vi "OCT with Classes.vi"() -> ()   [LabVIEW 2014]
doc: "I. Description:\nThis example demonstrates how to acquire a continuous amount of data (Waveform) using the DAQ device's internal clock.\n\nII. Instructions for Running:\n1. Create an analog input voltage channel.\n2. Set the rate for the sample clock. Additionally, define the sample mode to be continuous.\n3. Call the Start VI to start the acquisition.\n4. Read the waveform data in a loop until the user hits the stop button or an error occurs.\nNote: This example reads data from one or more channels and returns an array of data. Use the Index Array function to access an individual channel of data.\n5. Call the Clear Task VI to clear the Task.\n6. Use the popup dialog box to display an error if any.\n\nIV. I/O Connections Overview:\nMake sure your signal input terminal matches the Physical Channel I/O Control. For further connection information, refer to your hardware reference manual."
uses:
  Type Defs/OCT DAQ Channel Data Type.ctl
  Type Defs/OCT Hardware States.ctl
  Classes/Galvo/Scanning Cluster.ctl
  Classes/UT OCT Classes.ctl
  Classes/DAQ/ATS660/ATS660 Class.lvclass
  Classes/Galvo/NI Galvo/NI Galvo.lvclass
  Processing Class/Intensity/Intensity Processing.lvclass
  Classes/Laser/Santec/Santec.lvclass
  Classes/DAQ Control Functional Global States.ctl
  Signal Processing/Display Raw Data states.ctl
  DAQ Status States.ctl
  Signal Processing/processing_states.ctl
  Classes/Galvo/Galvo.lvclass
panel:
  out "Single A-Scan":u16[](graph)
  in  "Scanning Parameters":T1={"Fast Axis Offset"=0.0, "Slow Axis Offset"=0.0, "Slow Axis Amp"=2.0, "Fast Axis Amp"=2.0, "Scan Pattern"=enum."Raster"} {"Fast Axis Amp" max=20 format="%#.2f"; "Slow Axis Amp" max=20 format="%#.2f"; "Slow Axis Offset" max=10 format="%#.2f"; "Fast Axis Offset" max=10 format="%#.2f"}
  out "Log10?":bool
  in  "OCT Hardware States":T2
  out "Background Array":u16[](array[numeric])
  in  "Calibrate":bool
  in  "Save Sweep Button":bool
  in  "Data Format":T3
  in  "Save Sweep":bool
  in  "Stop Button":bool
  out "B-Scans Per Buffer":i32=1
  out "Clock Length":u32=9184
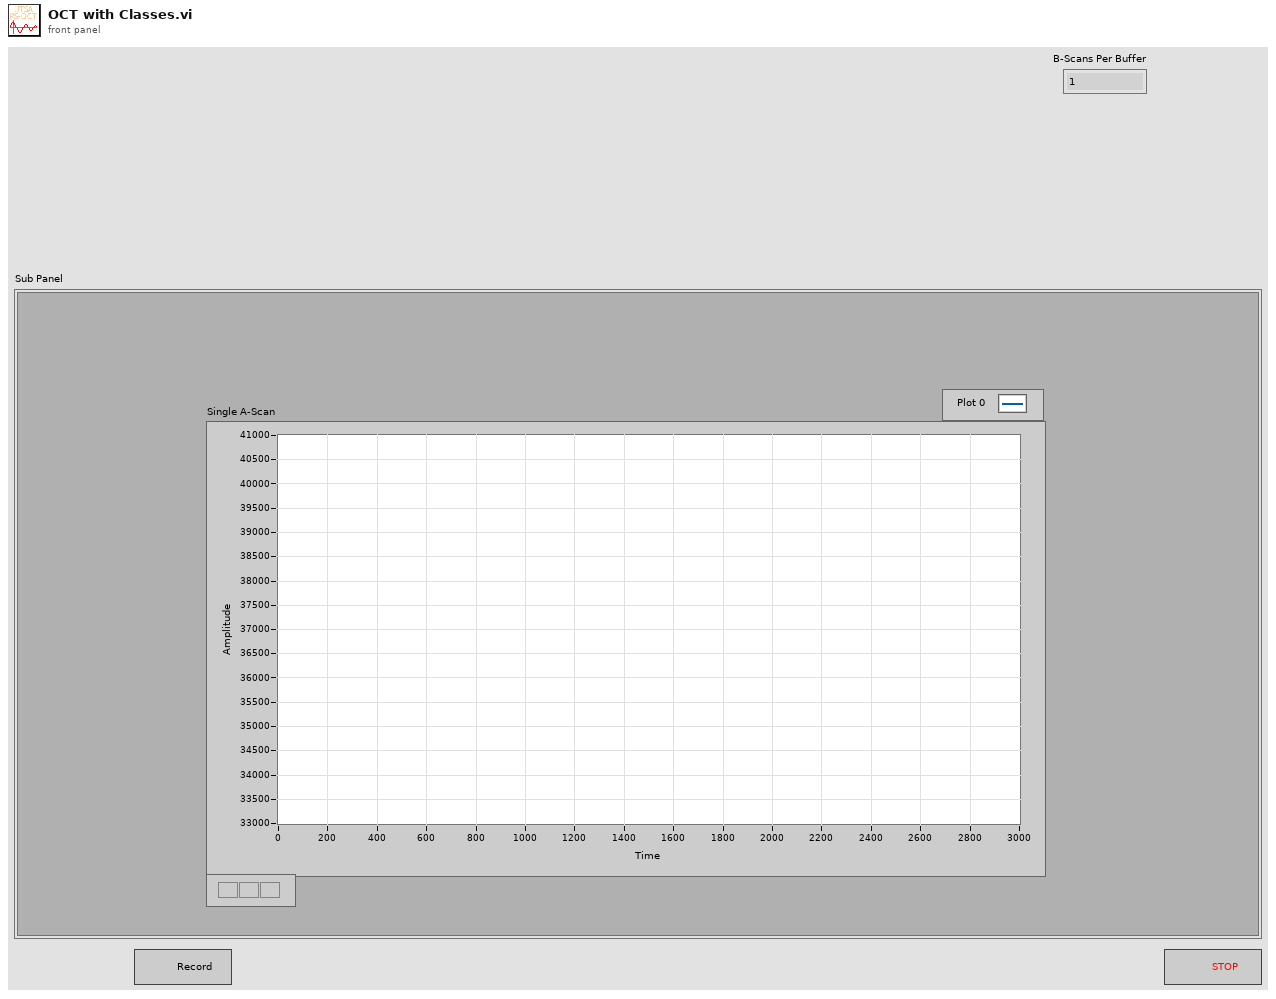
[diagram p1: front panel]
types:
  T1 = typedef "Galvo.lvclass/Scanning Cluster.ctl" = cluster{"Fast Axis Offset":sgl, "Slow Axis Offset":sgl, "Slow Axis Amp":sgl, "Fast Axis Amp":sgl, "Scan Pattern":enum16{"Raster"}}
  T2 = typedef "OCT Hardware States.ctl" = enum16{"Acquire Data", "Initialize Galvos", "Startup", "Reset DAQ", "Background Subtraction", "Acquire Background", "Update DAQ Parameters", "Stop", "Set Clock", "Initialize DAQ", "Set Resampling Array", "Save Sweep", "Configure Laser"}
  T3 = typedef "OCT DAQ Channel Data Type.ctl" = enum16{"Channel 1", "Channel 2", "Channel 1 and 2"}
  T4 = typedef "UT OCT Classes.ctl" = refnum<class "ATS660 Class.lvclass">
  T5 = typedef "DAQ Control Functional Global States.ctl" = enum16{"Status", "Set Processing Finished", "Reset", "Clear", "Set DAQ Finished"}
  T6 = typedef "DAQ Class.lvclass/DAQ Parameters.ctl" = cluster{"Points Per Trigger":u32, "Triggers per Buffer":u32, "Number of Buffers":u32, "Buffers per Transfer":u32, "Trigger Voltage":sgl, "Trigger Source":T7, "Trigger Slope":T8, "Channel":T3, "Clock":T9, "Bits per Sample":dbl, "Range":dbl}
  T7 = typedef "DAQ Class.lvclass/Trigger Source.ctl" = enum16{"External", "Channel A", "Channel B"}
  T8 = typedef "DAQ Class.lvclass/Trigger Slope.ctl" = enum16{"Rising", "Falling"}
  T9 = typedef "DAQ Class.lvclass/Clock Control.ctl" = enum16{"Internal Clock", "External Clock"}
  T10 = typedef "Display Raw Data states.ctl" = enum16{"Add Raw", "Add Processed", "Show"}
  T11 = typedef "DAQ Status States.ctl" = enum16{"Get", "Show"}
  T12 = enum32{"Invalid", "Standard", "Closed", "Hidden", "Minimized", "Maximized"}
  T13 = typedef "processing_states.ctl" = enum16{"Initialize", "Set Background", "Update Imaging Parameters", "Get Queue", "Process Data", "Get Size", "Flush Data", "Set Reample Array", "Get Last Processed BScan", "Shutdown"}
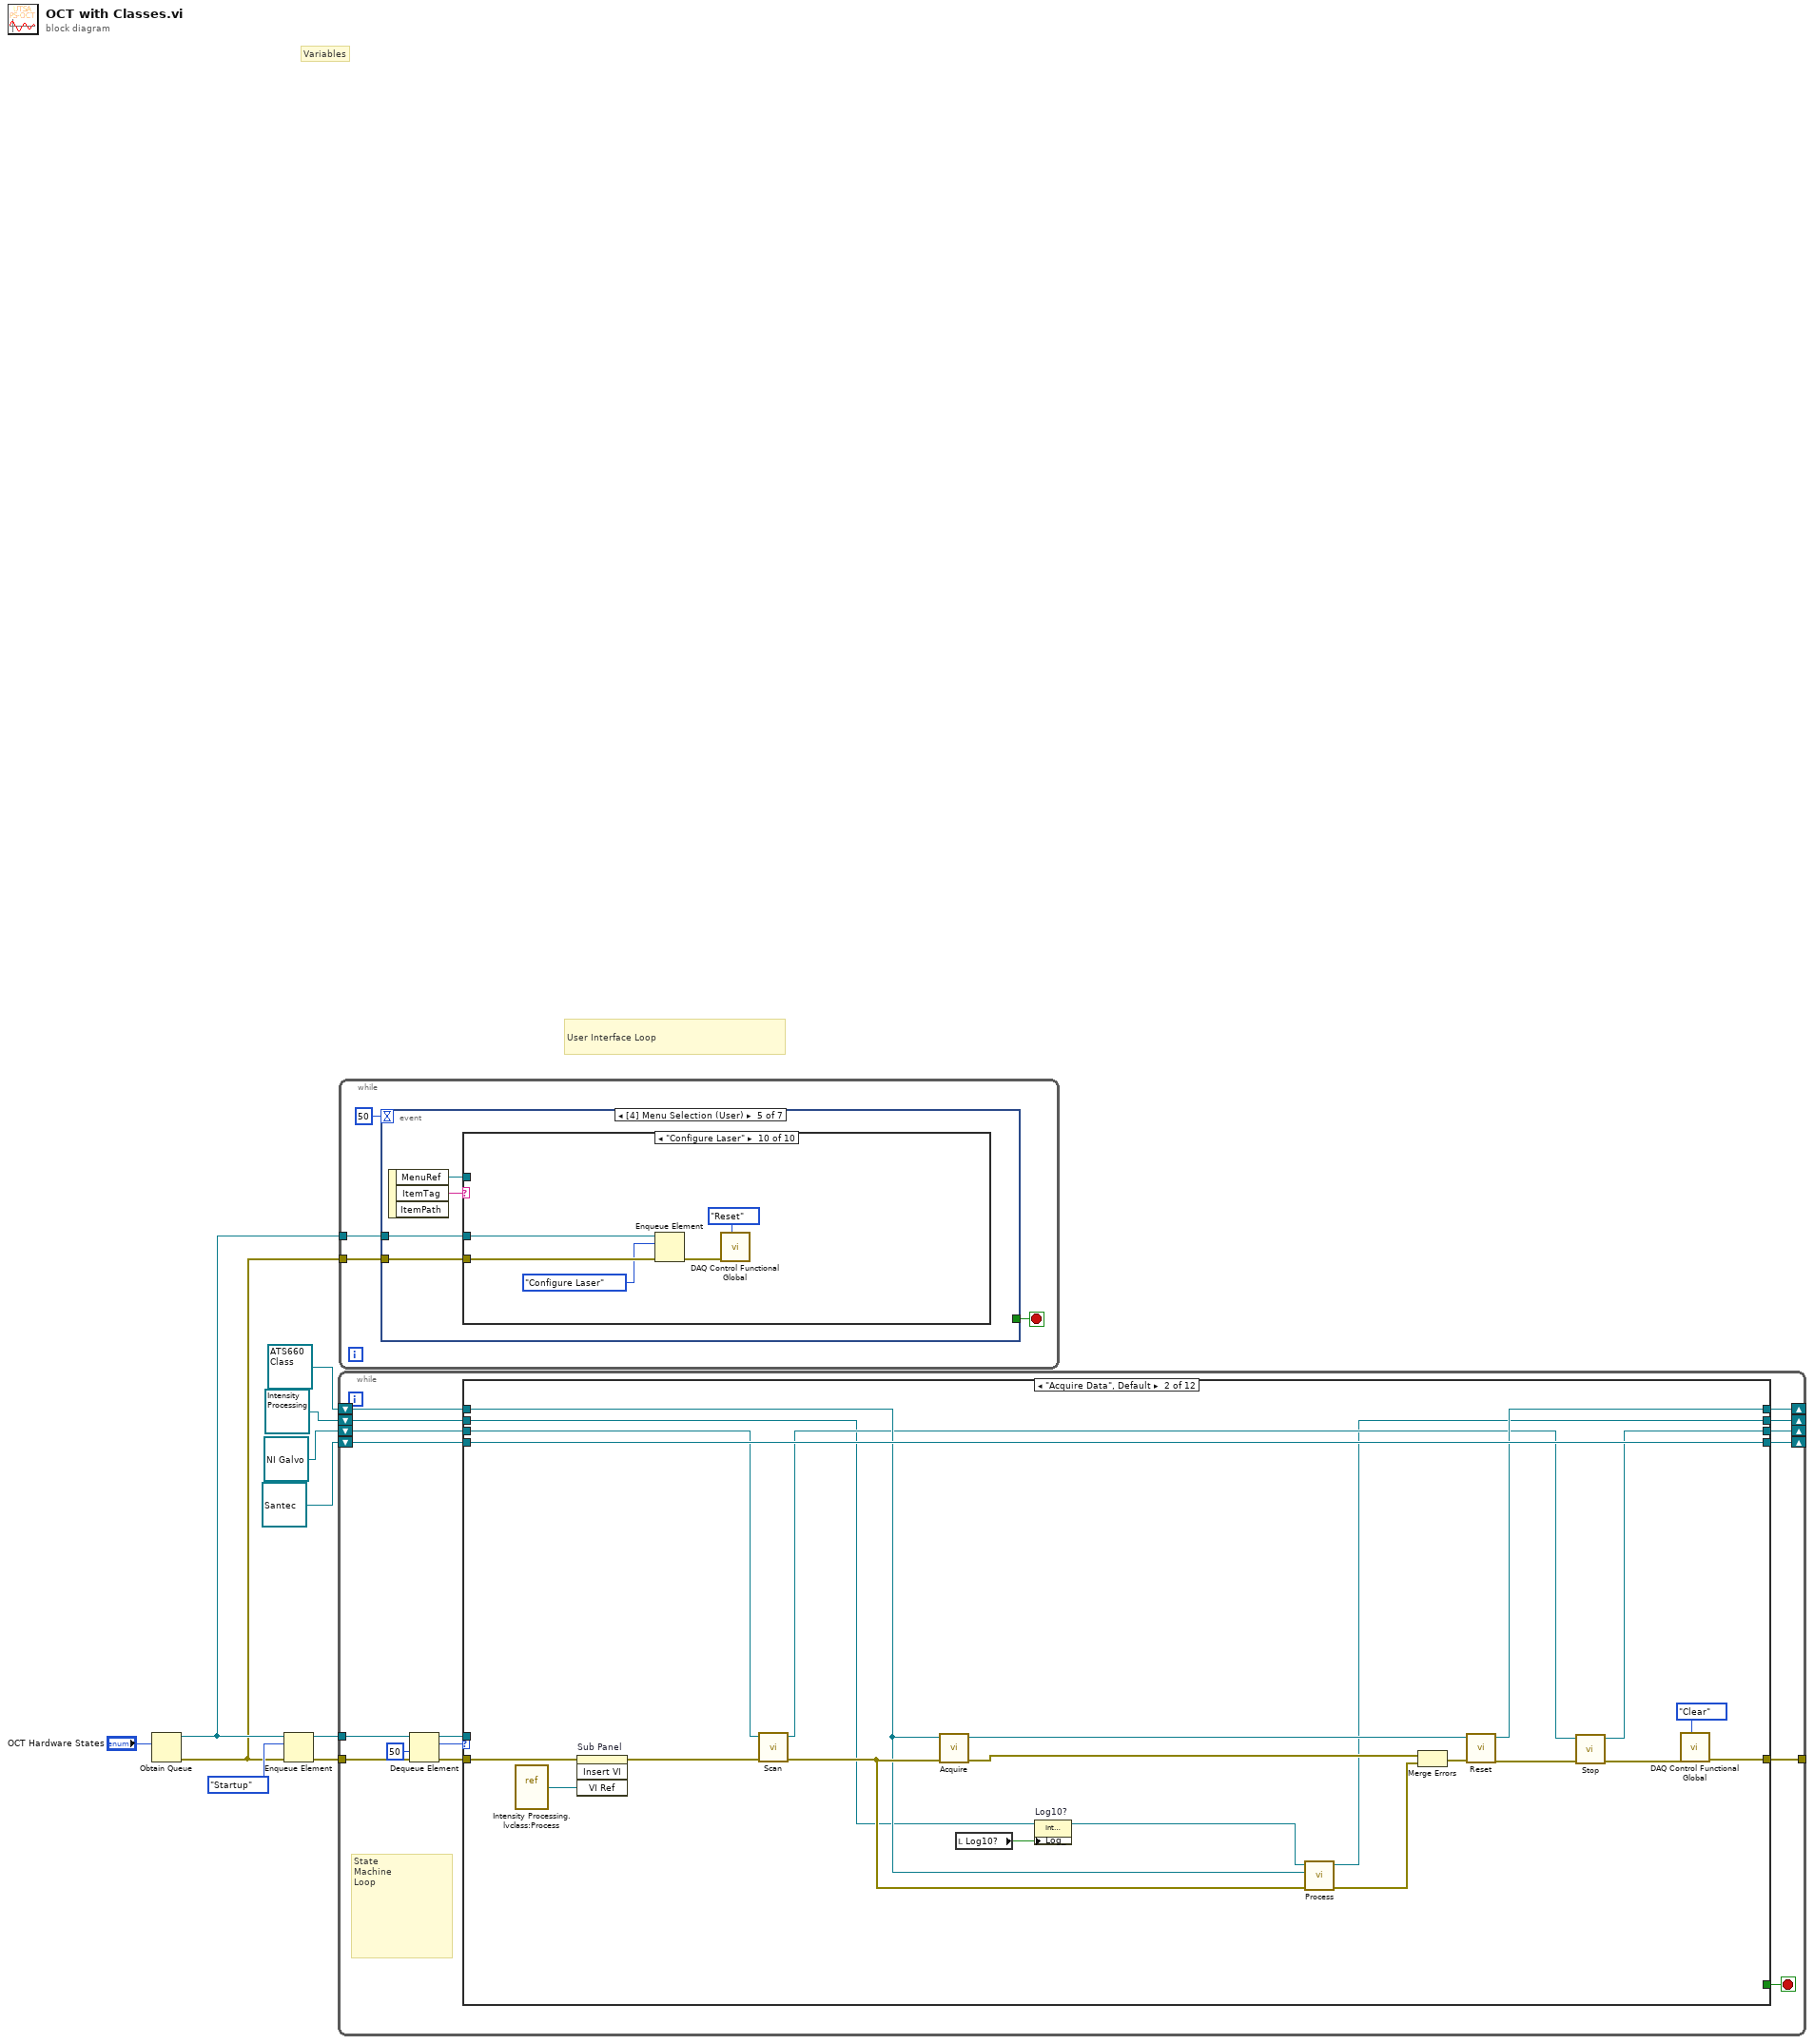
[diagram p0: block diagram]
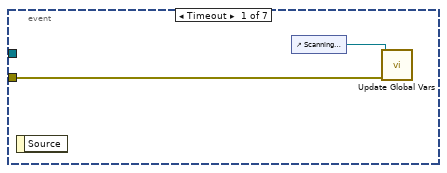
[diagram p2: hidden frame]
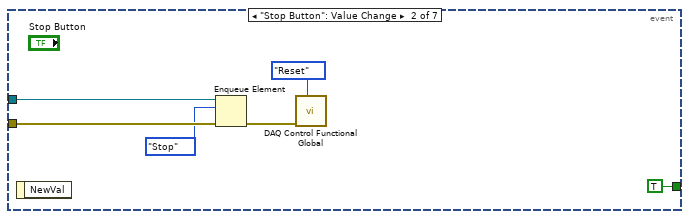
[diagram p3: hidden frame]
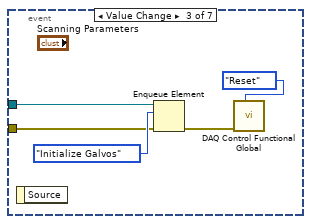
[diagram p4: hidden frame]
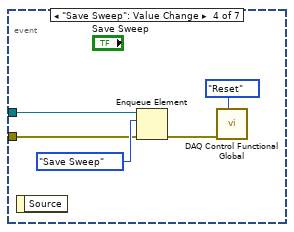
[diagram p5: hidden frame]
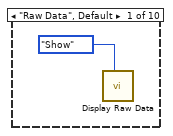
[diagram p6: hidden frame]
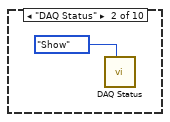
[diagram p7: hidden frame]
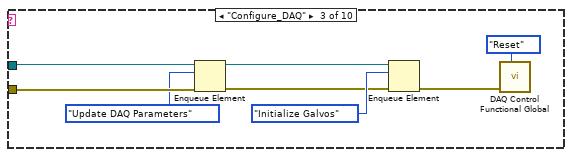
[diagram p8: hidden frame]
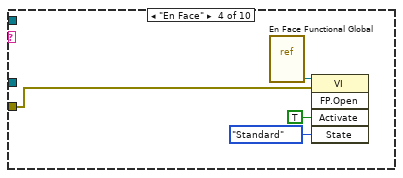
[diagram p9: hidden frame]
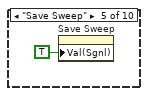
[diagram p10: hidden frame]
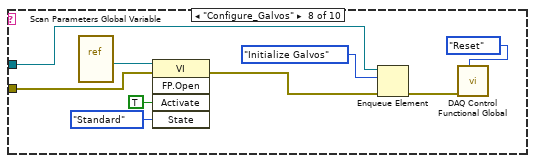
[diagram p13: hidden frame]
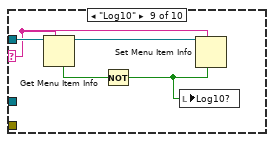
[diagram p14: hidden frame]
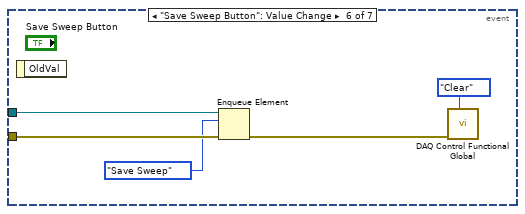
[diagram p15: hidden frame]
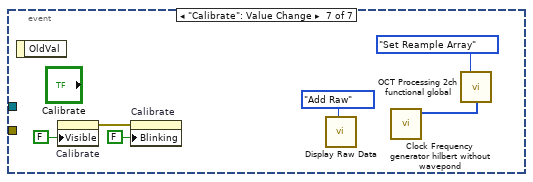
[diagram p16: hidden frame]
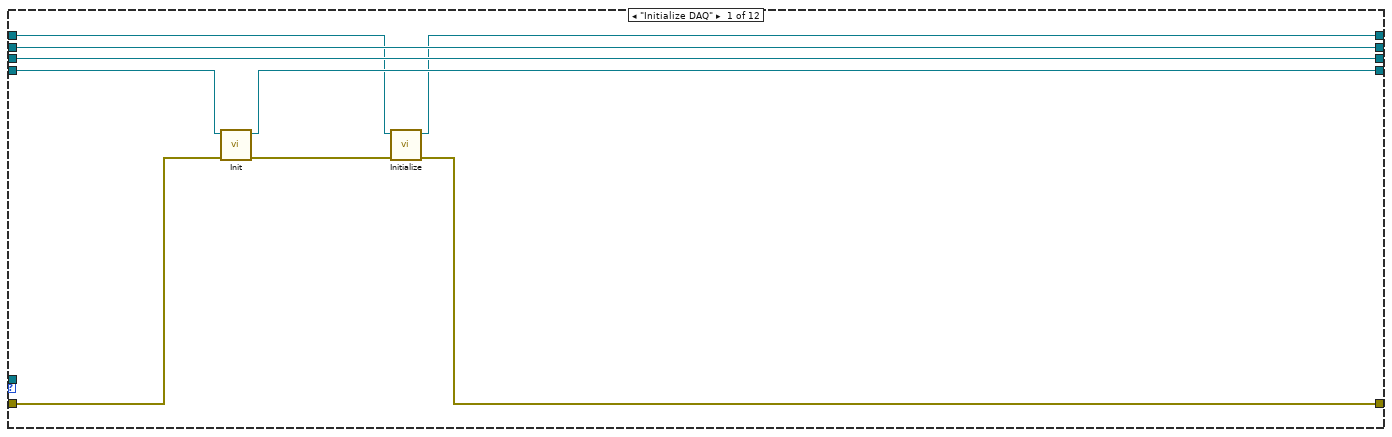
[diagram p17: hidden frame]
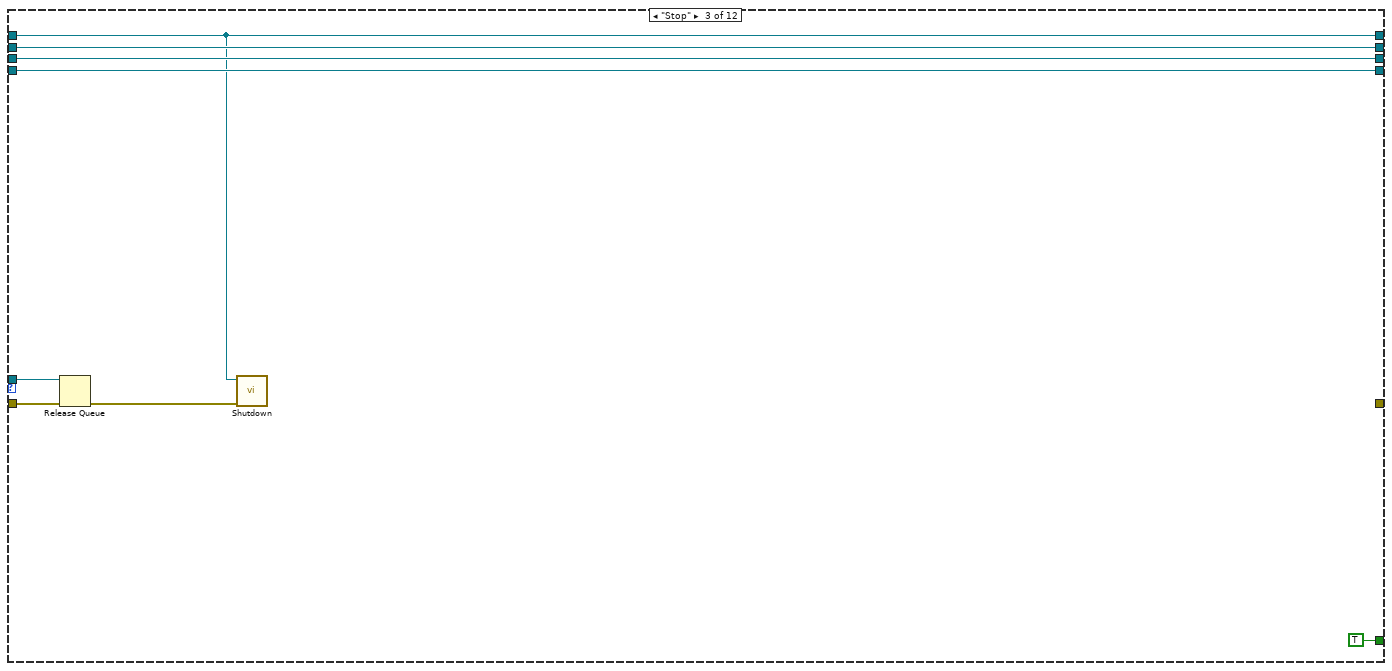
[diagram p18: hidden frame]
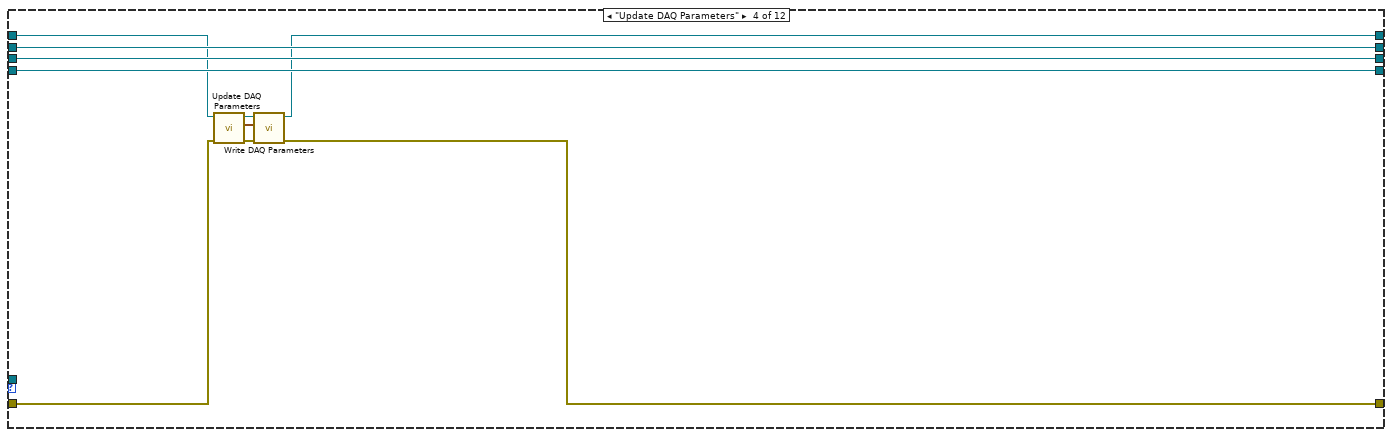
[diagram p19: hidden frame]
diagram:
  # "User Interface Loop"
  # "Variables"
  n1 = Obtain Queue(element data type="OCT Hardware States") -> (queue out=w8:refnum<queue>, error out=w5:errorcluster)  [unwired: 4 in, 1 out]
  n2 = Enqueue Element(queue=w8, element=OCT_Hardware_States."Startup", error in (no error)=w5) -> (queue out=w9:refnum<queue>, error out=w7:errorcluster)  [unwired: 1 in, 1 out]
  n3 = while {
    tunnel: w9 -> [w26]
    tunnel: w7 -> [w21]
    tunnel: [w22] -> _
    shift-right: [w18] -> _
    shift-left: T4 refnum ("ATS660 Class.lvclass") -> [w19]
    shift-right: [w14] -> _
    shift-left: refnum<class "Intensity Processing.lvclass"> refnum ("Intensity Processing.lvclass") -> [w17]
    shift-right: [w13] -> _
    shift-left: refnum<class "NI Galvo.lvclass"> refnum ("NI Galvo.lvclass") -> [w16]
    shift-right: [w12] -> _
    shift-left: refnum<class "Santec.lvclass"> refnum ("Santec.lvclass") -> [w15]
    stop <- w11 stop-if-true
    # "State\nMachine\nLoop"
    n4 = Dequeue Element(queue=w26, timeout in ms (-1)=50, error in (no error)=w21) -> (queue out=w24:refnum<queue>, element=w20:T2, error out=w25:errorcluster)  [unwired: 1 out]
    n5 = case shown="\"Acquire Data\", Default" w20 {
      tunnel: w25 -> [w34 w45 w64 w75 _ _ w98 _ w123 w137 w145 _]
      tunnel: w24 -> [_ _ w65 _ _ _ _ _ w124 w136 _ _]
      tunnel: [w35 w56 _ w71 _ _ w89 _ _ w134 w148 _] -> w22
      tunnel: w19 -> [w28 w41 w59 w67 w79 w83 w86 w105 w109 w133 w140 w155]
      tunnel: [w27 w40 w59 w66 w79 w83 w85 w105 w109 w132 w139 w155] -> w18
      tunnel: w17 -> [w32 w37 w62 w70 w78 w82 w88 w104 w108 w131 w144 w154]
      tunnel: w16 -> [w31 w42 w61 w69 w77 w81 w87 w103 w107 w130 w142 w153]
      tunnel: w15 -> [w30 w43 w60 w68 w76 w80 w84 w102 w106 w129 w143 w152]
      tunnel: [w32 w36 w62 w70 w78 w82 w88 w104 w108 w131 w144 w154] -> w14
      tunnel: [w31 w38 w61 w69 w77 w81 w87 w103 w107 w130 w141 w153] -> w13
      tunnel: [w29 w43 w60 w68 w76 w80 w84 w102 w106 w129 w143 w152] -> w12
      tunnel: [_ _ TRUE _ _ _ _ _ _ _ _ _] -> w11
      frame "Initialize DAQ" {
        n6 = call-dynamic "Init.vi"("error in (no error)"=w34, "Santec in"=w30) -> ("error out"=w33:errorcluster, "Santec out"=w29:refnum<class "Santec.lvclass">)  [unwired: 8 in]
        n7 = call-dynamic "Initialize.vi"("error in (no error)"=w33, "ATS660 Class in"=w28) -> ("error out"=w35:errorcluster, "ATS660 Class out"=w27:T4)  [unwired: 8 in]
      }
      frame "Acquire Data", Default {
        n8 = vi-ref "Intensity Processing.lvclass:Process.vi"() -> (w44:refnum<vi>)
        n9 = invoke on="Sub Panel" class="SubPanel" method="Insert VI"(error in=w45, "VI Ref"=w44) -> (error out=w49:errorcluster)  [unwired: 2 in, 3 out]
        n10 = call-dynamic "Scan.vi"("error in (no error)"=w49, "NI Galvo in"=w42) -> ("error out"=w48:errorcluster, "NI Galvo out"=w39:refnum<class "NI Galvo.lvclass">)  [unwired: 8 in]
        n11 = call-dynamic "Acquire.vi"("error in (no error)"=w48, "ATS660 Class in"=w41) -> ("error out"=w54:errorcluster, "ATS660 Class out"=w52:T4)  [unwired: 8 in]
        n12 = local read "Log10?"() -> (w50:bool)
        n13 = property on="Log10?" class="Intensity Processing.lvclass"(reference=w37, "Log_"=w50) -> (reference out=w51:refnum<class "Intensity Processing.lvclass">)  [unwired: 1 in, 1 out]
        n14 = call-dynamic "Process.vi"("error in (no error)"=w48, "DAQ Class.lvclass"=w41, "Intensity Processing in"=w51) -> ("error out"=w55:errorcluster, "Intensity Processing out"=w36:refnum<class "Intensity Processing.lvclass">)  [unwired: 7 in]
        n15 = Merge Errors(w54, w55) -> (w53:errorcluster)
        n16 = call-dynamic "Reset.vi"("error in (no error)"=w53, "ATS660 Class in"=w52) -> ("error out"=w47:errorcluster, "ATS660 Class out"=w40:T4)  [unwired: 8 in]
        n17 = call-dynamic "Stop.vi"("error in (no error)"=w47, "NI Galvo in"=w39) -> ("error out"=w46:errorcluster, "NI Galvo out"=w38:refnum<class "NI Galvo.lvclass">)  [unwired: 8 in]
        n18 = call "DAQ Control Functional Global.vi"("State"=DAQ_Control_Functional_Global_States."Clear", "Error In"=w46) -> ("Error Out"=w56:errorcluster)  [unwired: 6 in, 3 out]
      }
      frame "Stop" {
        n19 = Release Queue(queue=w65, error in (no error)=w64) -> (error out=w63:errorcluster)  [unwired: 1 in, 2 out]
        n20 = call-dynamic "Shutdown.vi"("error in (no error)"=w63, "ATS660 Class in"=w59) -> ()  [unwired: 8 in, 2 out]
      }
      frame "Update DAQ Parameters" {
        n21 = call-dynamic "Update DAQ Parameters.vi"("error in (no error)"=w75, "DAQ Class in"=w67) -> ("error out"=w73:errorcluster, "DAQ Parameters Out"=w72:T6, "DAQ Class out"=w74:T4)  [unwired: 7 in]
        n22 = call-dynamic "Write DAQ Parameters.vi"("error in (no error)"=w73, "DAQ Parameters"=w72, "ATS660 Class in"=w74) -> ("error out"=w71:errorcluster, "ATS660 Class out"=w66:T4)  [unwired: 7 in]
      }
      frame "Background Subtraction" {
      }
      frame "Acquire Background" {
      }
      frame "Set Clock" {
        n23 = call "DAQ Control Functional Global.vi"("State"=DAQ_Control_Functional_Global_States."Clear", "Error In"=w98) -> ("Error Out"=w97:errorcluster)  [unwired: 6 in, 3 out]
        n24 = call "Compute 1 A-Scan Parameters.vi"("error in (no error)"=w97, "Santec in"=w84, "ATS660 Class.lvclass in"=w86) -> ("error out"=w90:errorcluster, "DAQ Parameters"=w96:T6, "ATS660 Class out"=w91:T4)  [unwired: 6 in]
        n25 = call-dynamic "Write DAQ Parameters.vi"("error in (no error)"=w90, "DAQ Parameters"=w96, "ATS660 Class in"=w91) -> ("error out"=w95:errorcluster, "ATS660 Class out"=w94:T4)  [unwired: 7 in]
        n26 = call-dynamic "Reset.vi"("error in (no error)"=w95, "ATS660 Class in"=w94) -> ("error out"=w92:errorcluster, "ATS660 Class out"=w93:T4)  [unwired: 8 in]
        n27 = call-dynamic "Acquire.vi"("error in (no error)"=w92, "ATS660 Class in"=w93) -> ("error out"=w100:errorcluster, "ATS660 Class out"=w101:T4)  [unwired: 8 in]
        n28 = call-dynamic "Get Last Buffer.vi"("error in (no error)"=w100, "DAQ Class in"=w101) -> ("error out"=w89:errorcluster, "DAQ Class out"=w85:T4)  [unwired: 7 in, 1 out]
        n29 = call "Clock Frequency generator hilbert.vi"() -> ()  [unwired: 10 in, 2 out]
      }
      frame "Set Resampling Array" {
      }
      frame "Startup" {
        n30 = Enqueue Element(queue=w124, element=OCT_Hardware_States."Initialize DAQ", error in (no error)=w123) -> (queue out=w114:refnum<queue>, error out=w113:errorcluster)  [unwired: 1 in, 1 out]
        n31 = Enqueue Element(queue=w114, element=OCT_Hardware_States."Set Clock", error in (no error)=w113) -> (queue out=w112:refnum<queue>, error out=w111:errorcluster)  [unwired: 1 in, 1 out]
        n32 = Enqueue Element(queue=w112, element=OCT_Hardware_States."Update DAQ Parameters", error in (no error)=w111) -> (queue out=w126:refnum<queue>, error out=w125:errorcluster)  [unwired: 1 in, 1 out]
        n33 = local write "Stop Button"(FALSE ("Sweep Ready for saving")) -> ()
        n34 = Enqueue Element(queue=w126, element=OCT_Hardware_States."Initialize Galvos", error in (no error)=w125) -> (queue out=w117:refnum<queue>, error out=w116:errorcluster)  [unwired: 1 in, 1 out]
        n35 = Enqueue Element(queue=w117, element=OCT_Hardware_States."Acquire Data", error in (no error)=w116) -> ()  [unwired: 1 in, 3 out]
        "B-Scans Per Buffer" <- 4 ("B-Scans Per Buffer")
        "Clock Length" <- u32 9184 ("Clock Length")
        "Log10?" <- TRUE ("Log10?")
      }
      frame "Save Sweep" {
        n36 = Enqueue Element(queue=w136, element=OCT_Hardware_States."Acquire Data", error in (no error)=w137) -> (error out=w135:errorcluster)  [unwired: 1 in, 2 out]
        n37 = call-dynamic "Save.vi"("error in (no error)"=w135, "DAQ Class in"=w133) -> ("error out"=w134:errorcluster, "DAQ Class out"=w132:T4)  [unwired: 8 in]
      }
      frame "Initialize Galvos" {
        n38 = call-dynamic "Read DAQ Parameters.vi"("error in (no error)"=w145, "ATS660 Class in"=w140) -> ("error out"=w146:errorcluster, "DAQ Parameters"=w147:T6, "ATS660 Class out"=w139:T4)  [unwired: 7 in]
        n39 = local read "Scanning Parameters"() -> (w151:T1)
        n40 = call-dynamic "Configure.vi"("error in (no error)"=w146, "DAQ Parameters"=w147, "Scanning Parameters"=w151, "NI Galvo in"=w142) -> ("error out"=w150:errorcluster, "NI Galvo out"=w149:refnum<class "NI Galvo.lvclass">)  [unwired: 6 in]
        n41 = call-dynamic "Initialize.vi"("error in (no error)"=w150, "NI Galvo in"=w149) -> ("error out"=w148:errorcluster, "NI Galvo out"=w141:refnum<class "NI Galvo.lvclass">)  [unwired: 8 in]
      }
      frame "Reset DAQ" {
      }
    }
  }
  n42 = while {
    tunnel: w8 -> [w159]
    tunnel: w5 -> [w158]
    stop <- w156 stop-if-true
    n43 = event shown="[4] Menu Selection (User)" {
      selector: _ -> [_ _ _ _ _ _ _]
      dyn-events: _ -> [_ _ _ _ _ _ _]
      timeout: 50 -> [_ _ _ _ _ _ _]
      tunnel: w159 -> [_ w166 w169 w174 w180 w217 _]
      tunnel: w158 -> [w160 w167 w170 w175 w179 w219 _]
      tunnel: [_ TRUE _ _ _ _ _] -> w156
      event Timeout {
        n44 = event-data() -> ()  [unwired: 1 in, 1 out]
        n45 = control-ref of="Scanning Parameters"() -> (w161:refnum<vi>)
        n46 = call "Update Global Vars.vi"("Error In"=w160, "Cluster in"=w161) -> ()  [unwired: 9 in, 1 out]
      }
      event "Stop Button": Value Change {
        n47 = event-data() -> ()  [unwired: 1 in, 1 out]
        n48 = Enqueue Element(queue=w166, element=OCT_Hardware_States."Stop", error in (no error)=w167) -> (error out=w164:errorcluster)  [unwired: 1 in, 2 out]
        n49 = call "DAQ Control Functional Global.vi"("State"=DAQ_Control_Functional_Global_States."Reset", "Error In"=w164) -> ()  [unwired: 6 in, 4 out]
      }
      event Value Change {
        n50 = event-data() -> ()  [unwired: 1 in, 1 out]
        n51 = Enqueue Element(queue=w169, element=OCT_Hardware_States."Initialize Galvos", error in (no error)=w170) -> (error out=w171:errorcluster)  [unwired: 1 in, 2 out]
        n52 = call "DAQ Control Functional Global.vi"("State"=DAQ_Control_Functional_Global_States."Reset", "Error In"=w171) -> ()  [unwired: 6 in, 4 out]
      }
      event "Save Sweep": Value Change {
        n53 = event-data() -> ()  [unwired: 1 in, 1 out]
        n54 = Enqueue Element(queue=w174, element=OCT_Hardware_States."Save Sweep", error in (no error)=w175) -> (error out=w173:errorcluster)  [unwired: 1 in, 2 out]
        n55 = call "DAQ Control Functional Global.vi"("State"=DAQ_Control_Functional_Global_States."Reset", "Error In"=w173) -> ()  [unwired: 6 in, 4 out]
      }
      event Menu Selection (User) {
        n56 = event-data() -> ("MenuRef"=w178:refnum<k9>, "ItemTag"=w181:string)  [unwired: 1 in, 1 out]
        n57 = case shown="\"Configure Laser\"" w181 {
          selector: w181 -> [_ _ _ _ _ _ _ _ w207 _]
          tunnel: w180 -> [_ _ w191 _ _ _ _ w199 _ w215]
          tunnel: w179 -> [_ _ w190 w192 _ _ _ w197 _ w214]
          tunnel: w178 -> [_ _ _ _ _ _ _ _ w210 _]
          frame "Raw Data", Default {
            n58 = call "Display Raw Data.vi"("Enum"=Display_Raw_Data_states."Show") -> ()  [unwired: 11 in]
          }
          frame "DAQ Status" {
            n59 = call "DAQ Status.vi"("Enum"=DAQ_Status_States."Show") -> ()  [unwired: 9 in, 2 out]
          }
          frame "Configure_DAQ" {
            n60 = Enqueue Element(queue=w191, element=OCT_Hardware_States."Update DAQ Parameters", error in (no error)=w190) -> (queue out=w185:refnum<queue>, error out=w186:errorcluster)  [unwired: 1 in, 1 out]
            n61 = Enqueue Element(queue=w185, element=OCT_Hardware_States."Initialize Galvos", error in (no error)=w186) -> (error out=w184:errorcluster)  [unwired: 1 in, 2 out]
            n62 = call "DAQ Control Functional Global.vi"("State"=DAQ_Control_Functional_Global_States."Reset", "Error In"=w184) -> ()  [unwired: 6 in, 4 out]
          }
          frame "En Face" {
            n63 = vi-ref "En Face Functional Global.vi"() -> (w193:refnum<vi>)
            n64 = invoke class="VI" method="FP.Open"(reference=w193, error in=w192, "Activate"=TRUE ("Activate?"), "State"=T12."Standard") -> ()  [unwired: 1 in, 5 out]
          }
          frame "Save Sweep" {
            n65 = property on="Save Sweep" class="Bool (strict)"("Val(Sgnl)"=TRUE ("Value (Signaling)")) -> ()  [unwired: 2 in, 2 out]
          }
          frame "K-Space Correction" {
          }
          frame "Background Subtraction" {
          }
          frame "Configure_Galvos" {
            n66 = vi-ref "Scan Parameters Global Variable.vi"() -> (w205:refnum<vi>)
            n67 = invoke class="VI" method="FP.Open"(reference=w205, error in=w197, "Activate"=TRUE ("Activate?"), "State"=T12."Standard") -> (error out=w198:errorcluster)  [unwired: 1 in, 4 out]
            n68 = Enqueue Element(queue=w199, element=OCT_Hardware_States."Initialize Galvos", error in (no error)=w198) -> (error out=w201:errorcluster)  [unwired: 1 in, 2 out]
            n69 = call "DAQ Control Functional Global.vi"("State"=DAQ_Control_Functional_Global_States."Reset", "Error In"=w201) -> ()  [unwired: 6 in, 4 out]
          }
          frame "Log10" {
            n70 = Get Menu Item Info(7:w207, 11:w210) -> (3:w208:refnum<k9>, 4:w209:bool)  [unwired: 1 in, 5 out]
            n71 = Not(x=w209) -> (.not. x?=w206:bool)
            n72 = local write "Log10?"(w206) -> ()
            n73 = Set Menu Item Info(6:w206, 7:w207, 11:w208) -> ()  [unwired: 4 in, 2 out]
          }
          frame "Configure Laser" {
            n74 = Enqueue Element(queue=w215, element=OCT_Hardware_States."Configure Laser", error in (no error)=w214) -> (error out=w211:errorcluster)  [unwired: 1 in, 2 out]
            n75 = call "DAQ Control Functional Global.vi"("State"=DAQ_Control_Functional_Global_States."Reset", "Error In"=w211) -> ()  [unwired: 6 in, 4 out]
          }
        }
      }
      event "Save Sweep Button": Value Change {
        n76 = event-data() -> ()  [unwired: 1 in, 1 out]
        n77 = Enqueue Element(queue=w217, element=OCT_Hardware_States."Save Sweep", error in (no error)=w219) -> (error out=w218:errorcluster)  [unwired: 1 in, 2 out]
        n78 = call "DAQ Control Functional Global.vi"("State"=DAQ_Control_Functional_Global_States."Clear", "Error In"=w218) -> ()  [unwired: 6 in, 4 out]
      }
      event "Calibrate": Value Change {
        n79 = event-data() -> ()  [unwired: 1 in, 1 out]
        n80 = property on="Calibrate" class="Bool"("Visible"=FALSE) -> (error out=w225:errorcluster)  [unwired: 2 in, 1 out]
        n81 = property on="Calibrate" class="Bool"(error in=w225, "Blinking"=FALSE) -> ()  [unwired: 1 in, 2 out]
        n82 = call "Display Raw Data.vi"("Enum"=Display_Raw_Data_states."Add Raw") -> ()  [unwired: 11 in]
        n83 = call "Clock Frequency generator hilbert without wavepond.vi"() -> ("Zero Crossing Resample Index"=w221:i32[])  [unwired: 11 in]
        n84 = call "OCT Processing 2ch functional global.vi"("State"=processing_states."Set Reample Array", "Resample Array"=w221) -> ()  [unwired: 9 in, 5 out]
      }
    }
  }
